vi "Test Thermal Chamber Controller_DQMH API.vi"() -> ()   [LabVIEW 2015]
doc: "Thermal Chamber Controller_DQMH API Tester.\n____\nDelacor QMH Thermal Chamber Examples 4.0.0.21\nCopyright (c) 2018, Delacor"
uses:
  Heater State--enum.ctl
  Thermal Chamber Controller_DQMH.lvlib
panel:
  out "timed out?":bool
  in  "Refresh Button (sync)":bool
  in  "Refresh Button (asynchronous)":bool
  in  "Enable Heater":bool
  in  "Disable Heater":bool
  in  "Ramp Rate (deg C / second)":dbl=1.0
  in  "Temperature Set Point (deg C)":dbl=22.0
  out "Heater State":T1
  out "Actual Temperature":dbl format="%.2f"
  out "Furnace Temperature Chart":T2(graph)
  in  "Show Block Diagram":bool
  in  "Stop Module":bool
  in  "Start Module":bool
  in  "Hide Module Panel":bool
  in  "Show Module Panel":bool
  out "Status":string
  out "Module Running?":bool
  # "This VI tests the API for the Module."
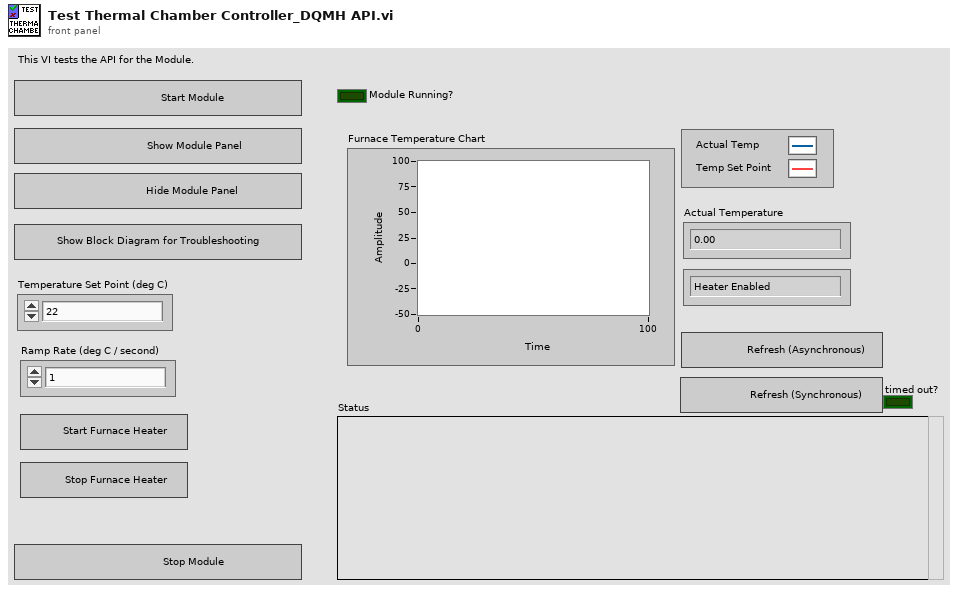
[diagram p1: front panel]
types:
  T1 = typedef "Thermal Chamber Controller_DQMH.lvlib/Heater State--enum.ctl" = enum16{"Heater Enabled", "Heater Disabled"}
  T2 = cluster{"Actual Temperature":dbl, "Required Temperature deg C":dbl}
  T3 = typedef "Thermal Chamber Controller_DQMH.lvlib/Broadcast Events--cluster.ctl" = cluster{"Module Did Init":refnum<user-event>, "Status Updated":refnum<user-event>, "Error Reported":refnum<user-event>, "Module Did Stop":refnum<user-event>, "Update Module Execution Status":refnum<user-event>, "Set Point Updated":refnum<user-event>, "Ramp Rate Updated":refnum<user-event>, "Heater State Updated":refnum<user-event>, "Chamber Status Updated":refnum<user-event>}
  T4 = cluster{"Actual Temperature":dbl, "Temperature Set Point":dbl}
  T5 = typedef "Thermal Chamber Controller_DQMH.lvlib/Request and Wait for Status (Reply Payload)--cluster.ctl" = cluster{"Actual Temperature":dbl, "Temperature Set Point":dbl, "Temperature Ramp Rate":dbl, "Heater State":T1, "error":errorcluster}
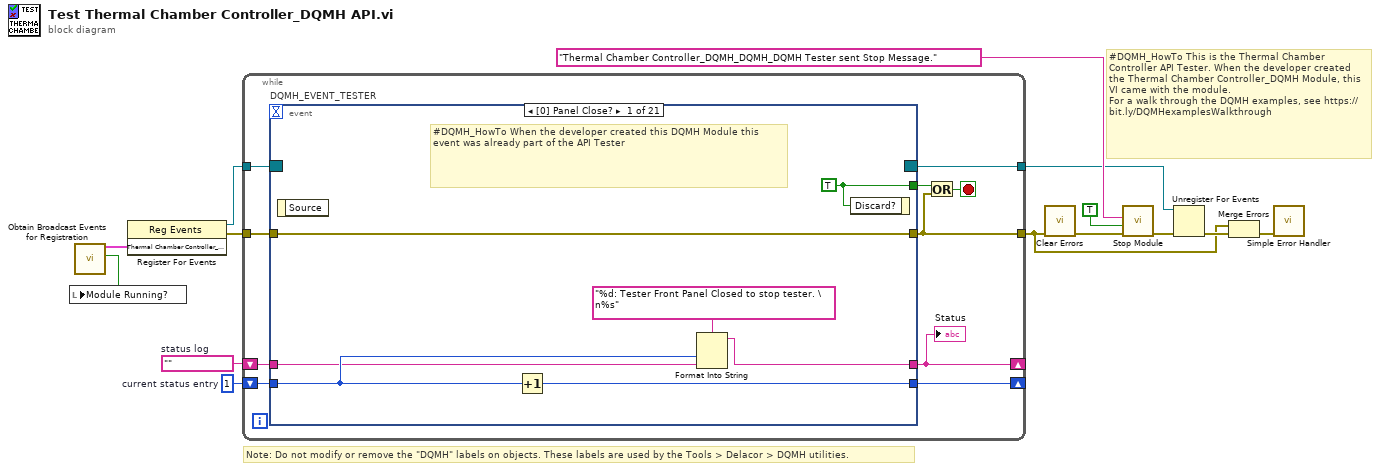
[diagram p0: block diagram]
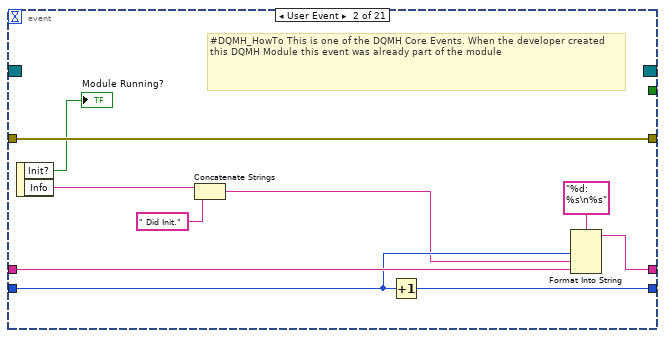
[diagram p2: hidden frame]
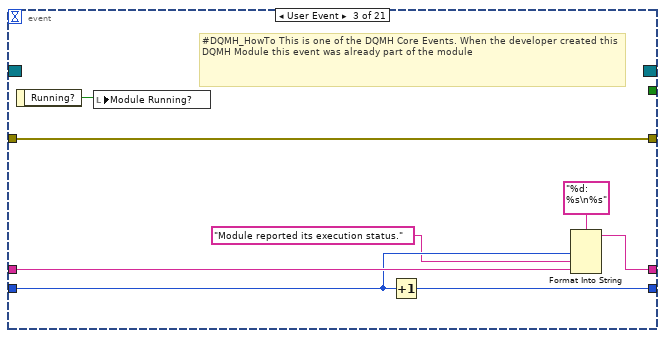
[diagram p3: hidden frame]
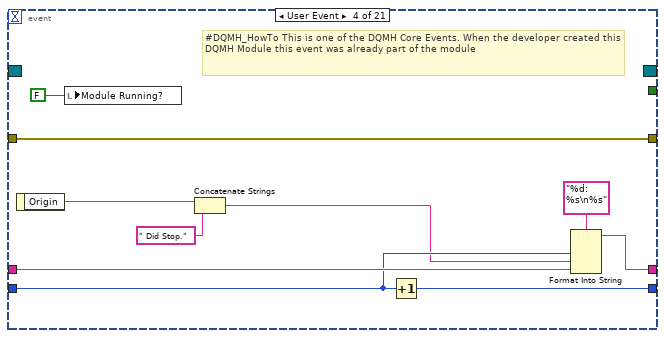
[diagram p4: hidden frame]
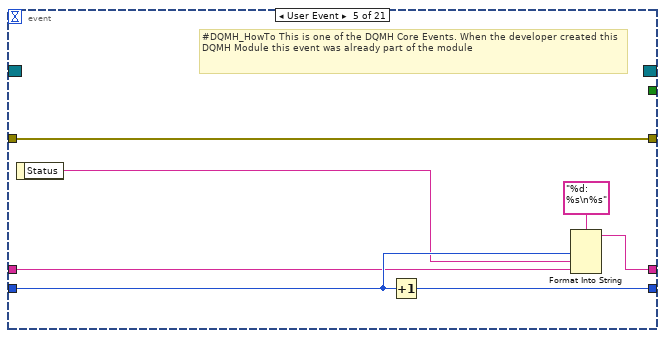
[diagram p5: hidden frame]
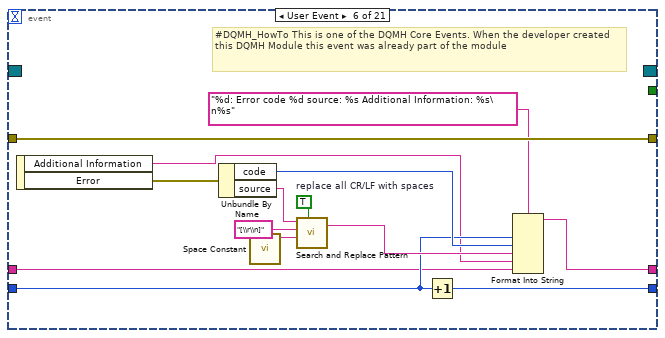
[diagram p6: hidden frame]
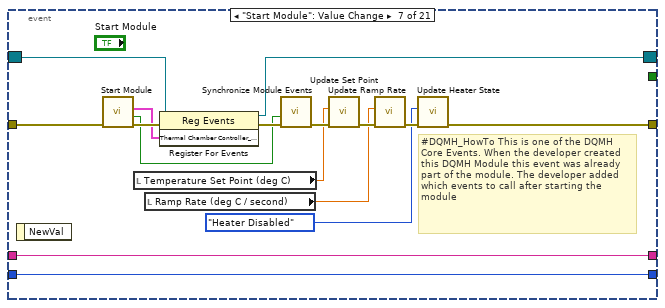
[diagram p7: hidden frame]
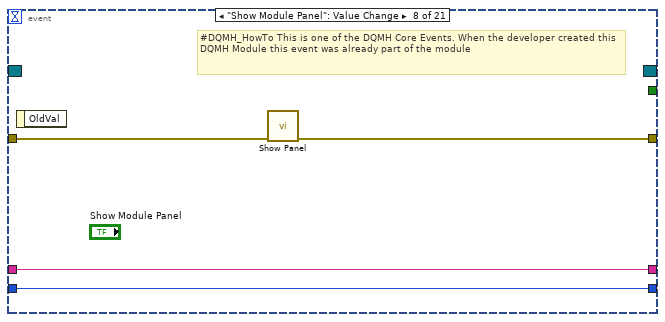
[diagram p8: hidden frame]
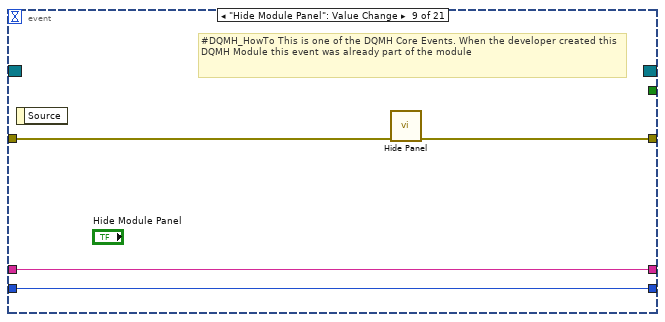
[diagram p9: hidden frame]
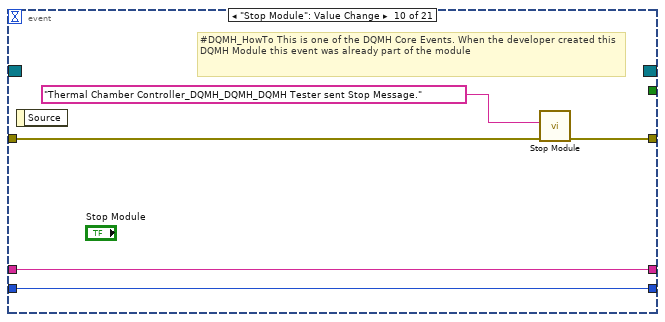
[diagram p10: hidden frame]
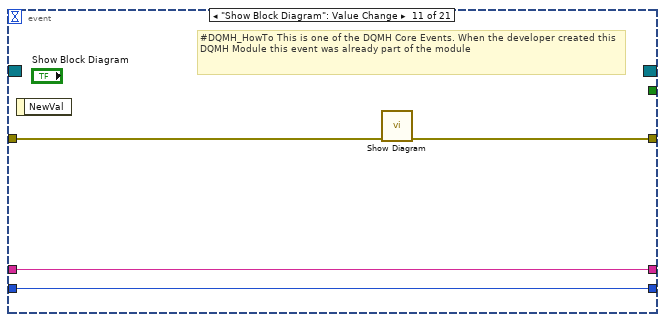
[diagram p11: hidden frame]
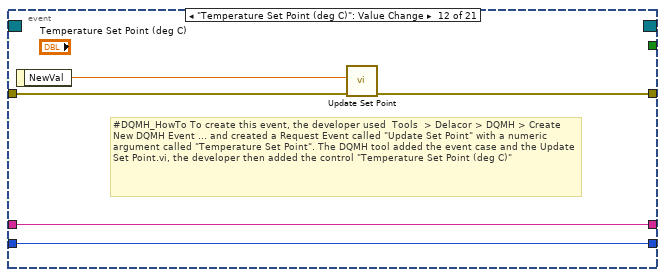
[diagram p12: hidden frame]
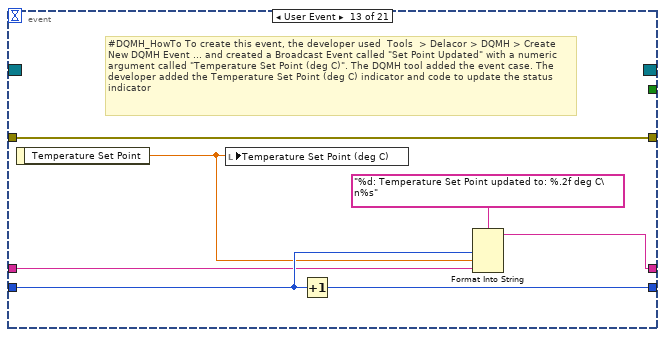
[diagram p13: hidden frame]
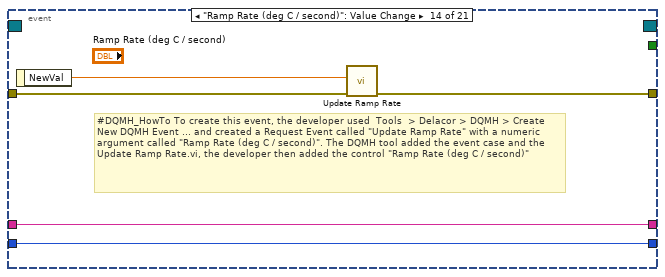
[diagram p14: hidden frame]
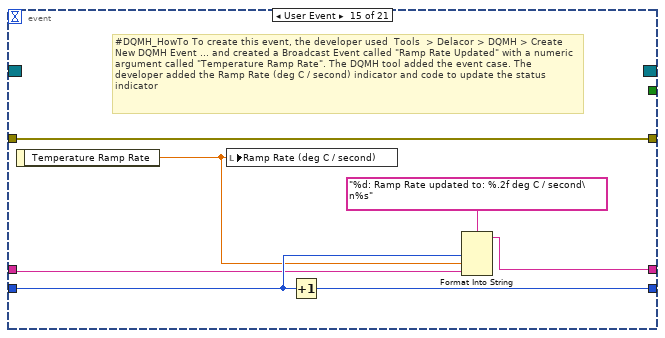
[diagram p15: hidden frame]
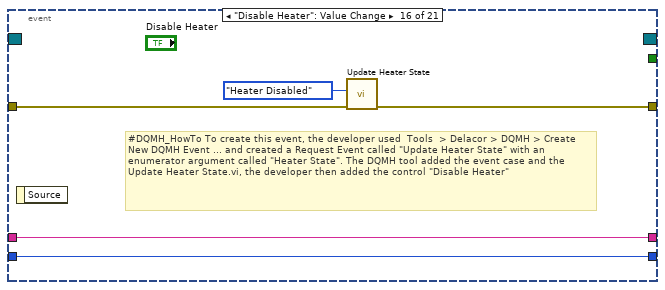
[diagram p16: hidden frame]
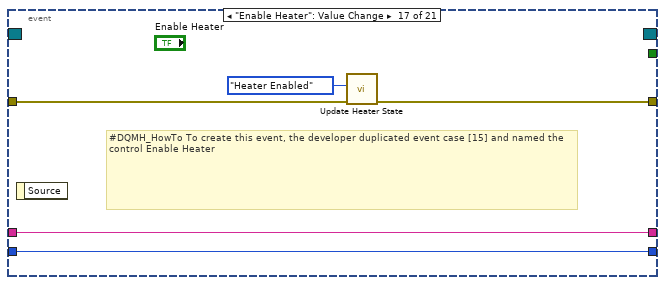
[diagram p17: hidden frame]
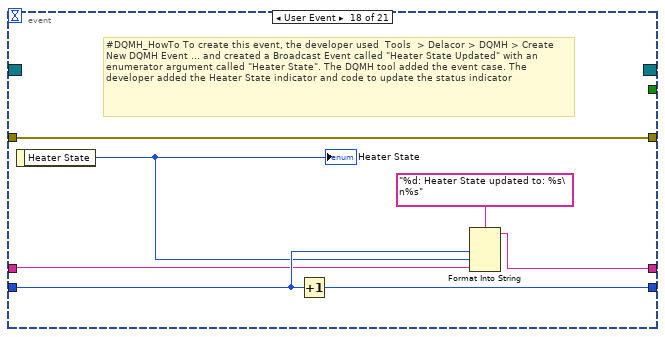
[diagram p18: hidden frame]
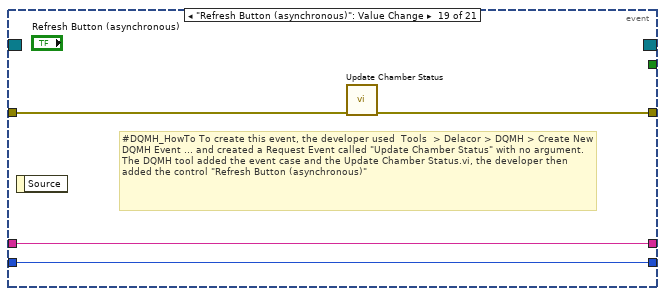
[diagram p19: hidden frame]
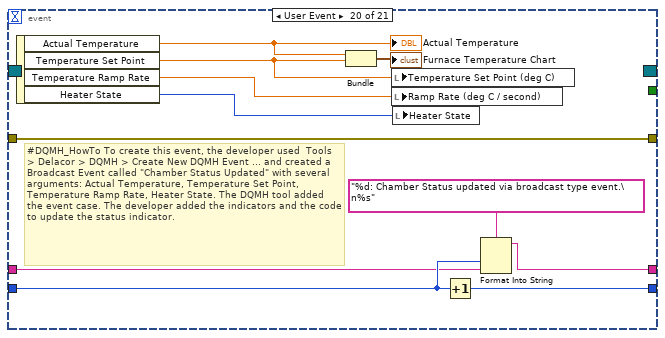
[diagram p20: hidden frame]
diagram:
  w10 = 1  # current status entry
  w11 = ""  # status log
  # "#DQMH_HowTo This is the Thermal Chamber Controller API Tester. When the developer created the Thermal Chamber Controller_DQMH Module, this VI came with the module.\nFor a walk through the DQMH examples, see https://bit.ly/DQMHexamplesWalkthrough"
  # "Note: Do not modify or remove the \"DQMH\" labels on objects. These labels are used by the Tools > Delacor > DQMH utilities."
  n1 = call "Obtain Broadcast Events for Registration.vi"() -> ("Already running?"=w4:bool, "Thermal Chamber Controller_DQMH Broadcast Events"=w8:T3)  [unwired: 9 in, 1 out]
  n2 = local write "Module Running?"(w4) -> ()
  n3 = register-events(w8) -> (reference out=w7:refnum<event-registration>, error out=w9:errorcluster)  [unwired: 2 in]
  n4 = while {
    tunnel: w7 -> [w24]
    tunnel: [w17] -> w1
    shift-right: [w19] -> _
    shift-left: w11 -> [w21]
    shift-right: [w20] -> _
    shift-left: w10 -> [w22]
    tunnel: w9 -> [w16]
    tunnel: [w15] -> w6
    stop <- w18 stop-if-true
    n5 = event "DQMH_EVENT_TESTER" shown="[0] Panel Close?" {
      selector: w24 -> [_ _ _ _ _ _ w90 _ _ _ _ _ _ _ _ _ _ _ _ _ _]
      dyn-events: [_ _ _ _ _ _ w89 _ _ _ _ _ _ _ _ _ _ _ _ _ _] -> w15
      timeout: _ -> [_ _ _ _ _ _ _ _ _ _ _ _ _ _ _ _ _ _ _ _ _]
      tunnel: [w31 _ _ _ _ _ _ _ _ _ _ _ _ _ _ _ _ _ _ _ _] -> w23
      tunnel: [w30 w41 w43 w50 w60 w80 w81 w100 w104 w107 w110 w115 w125 w127 w137 w139 w144 w154 w155 w169 w174] -> w17
      tunnel: w22 -> [w28 w37 w47 w57 w63 w70 w93 w98 w102 w108 w111 w116 w124 w128 w135 w140 w145 w152 w156 w162 w177]
      tunnel: w21 -> [w26 w38 w48 w58 w62 w68 w94 w99 w103 w109 w112 w117 w122 w129 w132 w141 w146 w148 w157 w159 w171]
      tunnel: [w25 w35 w45 w55 w64 w71 w94 w99 w103 w109 w112 w117 w121 w129 w133 w141 w146 w150 w157 w160 w172] -> w19
      tunnel: [w27 w36 w46 w56 w66 w69 w93 w98 w102 w108 w111 w116 w123 w128 w134 w140 w145 w151 w156 w161 w176] -> w20
      tunnel: w16 -> [w30 w41 w43 w50 w60 w80 w88 w97 w101 w105 w113 w118 w125 w130 w137 w142 w147 w154 w158 w169 w185]
      event Panel Close? {
        w31 = TRUE ("Discard?")
        # "#DQMH_HowTo When the developer created this DQMH Module this event was already part of the API Tester"
        n6 = event-data() -> ()  [unwired: 1 in, 1 out]
        n7 = Increment(x=w28) -> (x+1=w27:i32)
        n8 = Format Into String(format string="%d: Tester Front Panel Closed to stop tester. \n%s", w28, w26) -> (resulting string=w25:string)  [unwired: 2 in, 1 out]
        n9 = event-data("Discard?"=w31) -> ()  [unwired: 1 in, 1 out]
      }
      event User Event {
        # "#DQMH_HowTo This is one of the DQMH Core Events. When the developer created this DQMH Module this event was already part of the module"
        n10 = event-data() -> ("Init?"=→"Module Running?":bool, "Info"=w34:string)  [unwired: 1 in]
        n11 = Concatenate Strings(w34, " Did Init.") -> (w33:string)
        n12 = Increment(x=w37) -> (x+1=w36:i32)
        n13 = Format Into String(format string="%d: %s\n%s", w37, w33, w38) -> (resulting string=w35:string)  [unwired: 2 in, 1 out]
      }
      event User Event {
        # "#DQMH_HowTo This is one of the DQMH Core Events. When the developer created this DQMH Module this event was already part of the module"
        n14 = event-data() -> ("Running?"=w42:bool)  [unwired: 1 in]
        n15 = local write "Module Running?"(w42) -> ()
        n16 = Increment(x=w47) -> (x+1=w46:i32)
        n17 = Format Into String(format string="%d: %s\n%s", w47, "Module reported its execution status.", w48) -> (resulting string=w45:string)  [unwired: 2 in, 1 out]
      }
      event User Event {
        # "#DQMH_HowTo This is one of the DQMH Core Events. When the developer created this DQMH Module this event was already part of the module"
        n18 = event-data() -> ("Origin"=w54:string)  [unwired: 1 in]
        n19 = local write "Module Running?"(FALSE ("Module Did Init?")) -> ()
        n20 = Concatenate Strings(w54, " Did Stop.") -> (w53:string)
        n21 = Increment(x=w57) -> (x+1=w56:i32)
        n22 = Format Into String(format string="%d: %s\n%s", w57, w53, w58) -> (resulting string=w55:string)  [unwired: 2 in, 1 out]
      }
      event User Event {
        # "#DQMH_HowTo This is one of the DQMH Core Events. When the developer created this DQMH Module this event was already part of the module"
        n23 = event-data() -> ("Status"=w61:string)  [unwired: 1 in]
        n24 = Increment(x=w63) -> (x+1=w66:i32)
        n25 = Format Into String(format string="%d: %s\n%s", w63, w61, w62) -> (resulting string=w64:string)  [unwired: 2 in, 1 out]
      }
      event User Event {
        w76 = TRUE  # replace all CR/LF with spaces
        # "#DQMH_HowTo This is one of the DQMH Core Events. When the developer created this DQMH Module this event was already part of the module"
        n26 = event-data() -> ("Additional Information"=w67:string, "Error"=w72:errorcluster)  [unwired: 1 in]
        n27 = Unbundle By Name(w72) -> ("code"=w73:i32, "source"=w74:string)
        n28 = call <vilib>:"Space Constant.vi"() -> ("String"=w77:string)
        n29 = call <vilib>:"Search and Replace Pattern.vi"("string"=w74, "regular expression (\"\")"="[\\r\\n]" ("regular expression (\"\")"), "replace string (\"\")"=w77, "replace all? (F)"=w76) -> ("result string"=w75:string)  [unwired: 1 in, 1 out]
        n30 = Increment(x=w70) -> (x+1=w69:i32)
        n31 = Format Into String(format string="%d: Error code %d source: %s Additional Information: %s\n%s", w70, w73, w75, w67, w68) -> (resulting string=w71:string)  [unwired: 2 in, 1 out]
      }
      event "Start Module": Value Change {
        # "#DQMH_HowTo This is one of the DQMH Core Events. When the developer created this DQMH Module this event was already part of the module. The developer added which events to call after starting the module"
        n32 = event-data() -> ()  [unwired: 1 in, 1 out]
        n33 = call "Start Module.vi"("error in (no error)"=w88) -> ("error out"=w95:errorcluster, "Wait for Event Sync?"=w92:bool, "Thermal Chamber Controller_DQMH Broadcast Events"=w91:T3)  [unwired: 7 in, 1 out]
        n34 = local read "Temperature Set Point (deg C)"() -> (w86:dbl)
        n35 = local read "Ramp Rate (deg C / second)"() -> (w84:dbl)
        n36 = register-events(reference=w90, error in=w95, w91) -> (reference out=w89:refnum<event-registration>, error out=w96:errorcluster)
        n37 = call "Synchronize Module Events.vi"("error in (no error)"=w96, "Wait for Event Sync?"=w92) -> ("error out"=w87:errorcluster)  [unwired: 9 in]
        n38 = call "Update Set Point.vi"("error in (no error)"=w87, "Temperature Set Point"=w86) -> ("error out"=w85:errorcluster)  [unwired: 9 in]
        n39 = call "Update Ramp Rate.vi"("error in (no error)"=w85, "Temperature Ramp Rate"=w84) -> ("error out"=w83:errorcluster)  [unwired: 9 in]
        n40 = call "Update Heater State.vi"("error in (no error)"=w83, "Heater State"=Heater_State--enum."Heater Disabled") -> ("error out"=w81:errorcluster)  [unwired: 9 in]
      }
      event "Show Module Panel": Value Change {
        # "#DQMH_HowTo This is one of the DQMH Core Events. When the developer created this DQMH Module this event was already part of the module"
        n41 = event-data() -> ()  [unwired: 1 in, 1 out]
        n42 = call "Show Panel.vi"("error in (no error)"=w97) -> ("error out"=w100:errorcluster)  [unwired: 10 in]
      }
      event "Hide Module Panel": Value Change {
        # "#DQMH_HowTo This is one of the DQMH Core Events. When the developer created this DQMH Module this event was already part of the module"
        n43 = event-data() -> ()  [unwired: 1 in, 1 out]
        n44 = call "Hide Panel.vi"("error in (no error)"=w101) -> ("error out"=w104:errorcluster)  [unwired: 10 in]
      }
      event "Stop Module": Value Change {
        # "#DQMH_HowTo This is one of the DQMH Core Events. When the developer created this DQMH Module this event was already part of the module"
        n45 = event-data() -> ()  [unwired: 1 in, 1 out]
        n46 = call "Stop Module.vi"("error in (no error)"=w105, "Origin"="Thermal Chamber Controller_DQMH_DQMH_DQMH Tester sent Stop Message.") -> ("error out"=w107:errorcluster)  [unwired: 9 in]
      }
      event "Show Block Diagram": Value Change {
        # "#DQMH_HowTo This is one of the DQMH Core Events. When the developer created this DQMH Module this event was already part of the module"
        n47 = event-data() -> ()  [unwired: 1 in, 1 out]
        n48 = call "Show Diagram.vi"("error in (no error)"=w113) -> ("error out"=w110:errorcluster)  [unwired: 10 in]
      }
      event "Temperature Set Point (deg C)": Value Change {
        # "#DQMH_HowTo To create this event, the developer used  Tools  > Delacor > DQMH > Create New DQMH Event ... and created a Request Event called \"Update Set Point\" with a numeric argument called \"Temperature Set Point\". The DQMH tool added the event case and the Update Set Point.vi, the developer then added the control \"Temperature Set Point (deg C)\""
        n49 = event-data() -> ("NewVal"=w114:dbl)  [unwired: 1 in]
        n50 = call "Update Set Point.vi"("error in (no error)"=w118, "Temperature Set Point"=w114) -> ("error out"=w115:errorcluster)  [unwired: 9 in]
      }
      event User Event {
        # "#DQMH_HowTo To create this event, the developer used  Tools  > Delacor > DQMH > Create New DQMH Event ... and created a Broadcast Event called \"Set Point Updated\" with a numeric argument called \"Temperature Set Point (deg C)\". The DQMH tool added the event case. The developer added the Temperature Set Point (deg C) indicator and code to update the status indicator"
        n51 = event-data() -> ("Temperature Set Point"=w119:dbl)  [unwired: 1 in]
        n52 = local write "Temperature Set Point (deg C)"(w119) -> ()
        n53 = Increment(x=w124) -> (x+1=w123:i32)
        n54 = Format Into String(format string="%d: Temperature Set Point updated to: %.2f deg C\n%s", w124, w119, w122) -> (resulting string=w121:string)  [unwired: 2 in, 1 out]
      }
      event "Ramp Rate (deg C / second)": Value Change {
        # "#DQMH_HowTo To create this event, the developer used  Tools  > Delacor > DQMH > Create New DQMH Event ... and created a Request Event called \"Update Ramp Rate\" with a numeric argument called \"Ramp Rate (deg C / second)\". The DQMH tool added the event case and the Update Ramp Rate.vi, the developer then added the control \"Ramp Rate (deg C / second)\""
        n55 = event-data() -> ("NewVal"=w126:dbl)  [unwired: 1 in]
        n56 = call "Update Ramp Rate.vi"("error in (no error)"=w130, "Temperature Ramp Rate"=w126) -> ("error out"=w127:errorcluster)  [unwired: 9 in]
      }
      event User Event {
        # "#DQMH_HowTo To create this event, the developer used  Tools  > Delacor > DQMH > Create New DQMH Event ... and created a Broadcast Event called \"Ramp Rate Updated\" with a numeric argument called \"Temperature Ramp Rate\". The DQMH tool added the event case. The developer added the Ramp Rate (deg C / second) indicator and code to update the status indicator"
        n57 = event-data() -> ("Temperature Ramp Rate"=w131:dbl)  [unwired: 1 in]
        n58 = local write "Ramp Rate (deg C / second)"(w131) -> ()
        n59 = Increment(x=w135) -> (x+1=w134:i32)
        n60 = Format Into String(format string="%d: Ramp Rate updated to: %.2f deg C / second\n%s", w135, w131, w132) -> (resulting string=w133:string)  [unwired: 2 in, 1 out]
      }
      event "Disable Heater": Value Change {
        # "#DQMH_HowTo To create this event, the developer used  Tools  > Delacor > DQMH > Create New DQMH Event ... and created a Request Event called \"Update Heater State\" with an enumerator argument called \"Heater State\". The DQMH tool added the event case and the Update Heater State.vi, the developer then added the control \"Disable Heater\""
        n61 = event-data() -> ()  [unwired: 1 in, 1 out]
        n62 = call "Update Heater State.vi"("error in (no error)"=w142, "Heater State"=Heater_State--enum."Heater Disabled") -> ("error out"=w139:errorcluster)  [unwired: 9 in]
      }
      event "Enable Heater": Value Change {
        # "#DQMH_HowTo To create this event, the developer duplicated event case [15] and named the control Enable Heater"
        n63 = event-data() -> ()  [unwired: 1 in, 1 out]
        n64 = call "Update Heater State.vi"("error in (no error)"=w147, "Heater State"=Heater_State--enum."Heater Enabled") -> ("error out"=w144:errorcluster)  [unwired: 9 in]
      }
      event User Event {
        # "#DQMH_HowTo To create this event, the developer used  Tools  > Delacor > DQMH > Create New DQMH Event ... and created a Broadcast Event called \"Heater State Updated\" with an enumerator argument called \"Heater State\". The DQMH tool added the event case. The developer added the Heater State indicator and code to update the status indicator"
        n65 = event-data() -> ("Heater State"=w149:T1)  [unwired: 1 in]
        "Heater State" <- w149
        n66 = Increment(x=w152) -> (x+1=w151:i32)
        n67 = Format Into String(format string="%d: Heater State updated to: %s\n%s", w152, w149, w148) -> (resulting string=w150:string)  [unwired: 2 in, 1 out]
      }
      event "Refresh Button (asynchronous)": Value Change {
        # "#DQMH_HowTo To create this event, the developer used  Tools  > Delacor > DQMH > Create New DQMH Event ... and created a Request Event called \"Update Chamber Status\" with no argument. The DQMH tool added the event case and the Update Chamber Status.vi, the developer then added the control \"Refresh Button (asynchronous)\""
        n68 = event-data() -> ()  [unwired: 1 in, 1 out]
        n69 = call "Update Chamber Status.vi"("error in (no error)"=w158) -> ("error out"=w155:errorcluster)  [unwired: 10 in]
      }
      event User Event {
        # "#DQMH_HowTo To create this event, the developer used  Tools  > Delacor > DQMH > Create New DQMH Event ... and created a Broadcast Event called \"Chamber Status Updated\" with several arguments: Actual Temperature, Temperature Set Point, Temperature Ramp Rate, Heater State. The DQMH tool added the event case. The developer added the indicators and the code to update the status indicator."
        n70 = event-data() -> ("Actual Temperature"=w167:dbl, "Temperature Set Point"=w168:dbl, "Temperature Ramp Rate"=w166:dbl, "Heater State"=w164:T1)  [unwired: 1 in]
        "Actual Temperature" <- w167
        n71 = Bundle("Actual Temperature"=w167, "Temperature Set Point"=w168) -> (→"Furnace Temperature Chart":T4)  [unwired: 1 in]
        n72 = local write "Temperature Set Point (deg C)"(w168) -> ()
        n73 = local write "Ramp Rate (deg C / second)"(w166) -> ()
        n74 = local write "Heater State"(w164) -> ()
        n75 = Increment(x=w162) -> (x+1=w161:i32)
        n76 = Format Into String(format string="%d: Chamber Status updated via broadcast type event.\n%s", w162, w159) -> (resulting string=w160:string)  [unwired: 2 in, 1 out]
      }
      event "Refresh Button (sync)": Value Change {
        # "#DQMH_HowTo To create this event, the developer used  Tools  > Delacor > DQMH > Create New DQMH Event ... and created a Request and Wait for Reply Event called \"Request and Wait for Status\". The DQMH Tool added the event case and the Request and Wait for Status.vi"
        # "Only update status if there was no error or timeout from the method call"
        n77 = event-data() -> ()  [unwired: 1 in, 1 out]
        n78 = call "Request and Wait for Status.vi"("error in (no error)"=w185) -> ("error out"=w174:errorcluster, "timed out?"=w175:bool, "Reply Payload"=w184:T5)  [unwired: 8 in]
        "timed out?" <- w175
        n79 = Unbundle By Name(w184) -> ("Actual Temperature"=w183:dbl, "Temperature Set Point"=w182:dbl, "Temperature Ramp Rate"=w179:dbl, "Heater State"=w180:T1)
        n80 = Increment(x=w177) -> (x+1=w176:i32)
        n81 = Compound Arithmetic op=AND(invert w174, invert w175) -> (w170:bool)
        n82 = Bundle("Actual Temperature"=w183, "Temperature Set Point"=w182) -> (w181:T4)  [unwired: 1 in]
        n83 = Format Into String(format string="%d: Chamber Status updated via Request and Wait for Reply type event. \n%s", w177, w171) -> (resulting string=w173:string)  [unwired: 2 in, 1 out]
        n84 = local write "Actual Temperature"(w183) -> ()
        n85 = local write "Furnace Temperature Chart"(w181) -> ()
        n86 = local write "Temperature Set Point (deg C)"(w182) -> ()
        n87 = local write "Ramp Rate (deg C / second)"(w179) -> ()
        n88 = local write "Heater State"(w180) -> ()
        n89 = Select(t=w173, s=w170, f=w171) -> (s? t:f=w172:string)
      }
    }
    "Status" <- w19
    n90 = Or(x=w23, y=w17) -> (x .or. y?=w18:bool)
  }
  n91 = call <vilib>:"Clear Errors.vi"("error in (no error)"=w1) -> ("error out"=w3:errorcluster)  [unwired: 5 in, 1 out]
  n92 = call "Stop Module.vi"("error in (no error)"=w3, "Wait for Module to Stop? (F)"=TRUE ("Wait for Module to stop?"), "Origin"="Thermal Chamber Controller_DQMH_DQMH_DQMH Tester sent Stop Message.") -> ("error out"=w13:errorcluster)  [unwired: 8 in]
  n93 = Unregister For Events(event registration refnum=w6, error in=w13) -> (error out=w14:errorcluster)
  n94 = Merge Errors(w1, w14) -> (w2:errorcluster)
  n95 = call <vilib>:"Simple Error Handler.vi"("error in (no error)"=w2) -> ()  [unwired: 4 in, 5 out]
